vi "Initiate TS.vi"(8 "error in":errorcluster, 11 "Test Stand in":refnum<class "Cryo Sep Test Stand.lvclass">) -> (0 "error out":errorcluster, 3 "Test Stand out":refnum<class "Cryo Sep Test Stand.lvclass">)   [LabVIEW 2019, in "Test Stands.lvlib" / "Cryo Sep Test Stand.lvclass"]
uses:
  Cryo Sep Test Stand.lvclass
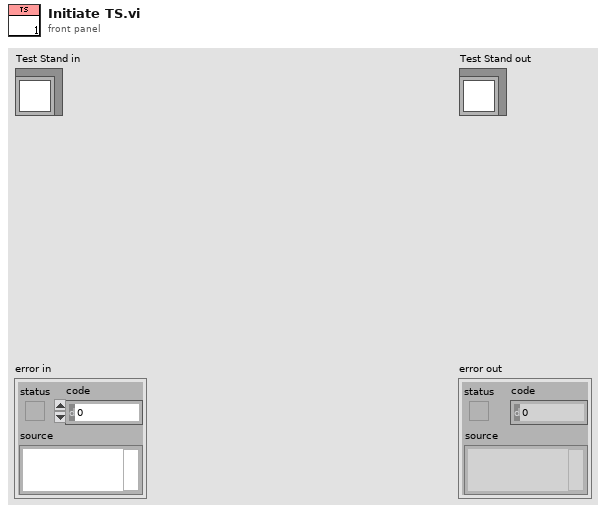
[diagram p1: front panel]
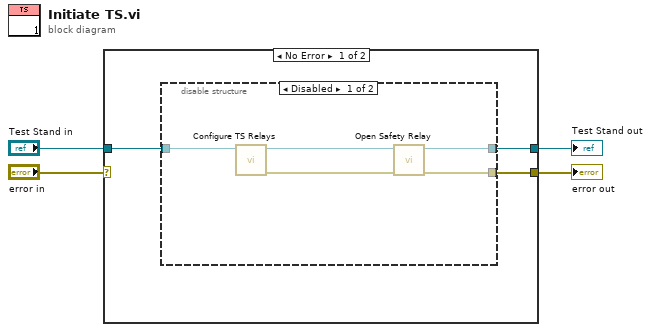
[diagram p0: block diagram]
diagram:
  n1 = case shown="No Error" "error in" {
    selector: "error in" -> [_ w15]
    tunnel: [w5 w15] -> w4
    tunnel: [w6 w14] -> w3
    tunnel: "Test Stand in" -> [w7 w14]
    frame No Error {
      n2 = disable-structure shown="Disabled" {
        disable-tunnel: w7 -> [w12 w13]
        disable-tunnel: [w10 w13] -> w6
        disable-tunnel: [w8 _] -> w5
        frame Disabled {
          n3 = call "Configure TS Relays.vi"("Test Stand in"=w12) -> ("error out"=w9:errorcluster, "Test Stand out"=w11:refnum<class "Cryo Sep Test Stand.lvclass">)  [unwired: 9 in]
          n4 = call "Open Safety Relay.vi"("error in (no error)"=w9, "Test Stand in"=w11) -> ("error out"=w8:errorcluster, "Test Stand out"=w10:refnum<class "Cryo Sep Test Stand.lvclass">)  [unwired: 8 in]
        }
        frame Enabled {
        }
      }
    }
    frame Error {
    }
  }
  "error out" <- w4
  "Test Stand out" <- w3
